vi "CSM - Synchronized Call.vi"   [LabVIEW 2017, in "CSM-QuickDrops.lvlib"]
doc: "Code snippet for calling a CSM module synchronously. This VI calls CSM module directly as a subVI.\n\n<b>Reference Example</b>: `[CSM-Example]\\2. Caller is CSM Scenario\\CSM Example - Caller is a CSM.vi`."
uses:
  CSM-QuickDrops.lvlib
  Communicable State Machine.lvlib
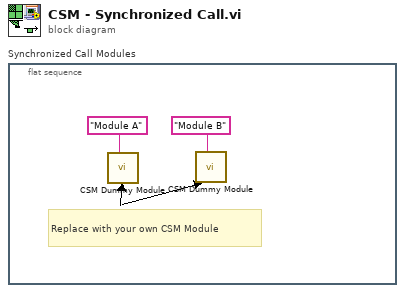
[diagram p0: block diagram]
diagram:
  n1 = flat-sequence "Synchronized Call Modules" {
    frame #0 {
      # "Replace with your own CSM Module"
      n2 = call "CSM Dummy Module.vi"("Name (\"\" to Use UUID)"="Module A" ("Name (\"\" to Use UUID)")) -> ()  [unwired: 11 in]
      n3 = call "CSM Dummy Module.vi"("Name (\"\" to Use UUID)"="Module B" ("Name (\"\" to Use UUID)")) -> ()  [unwired: 11 in]
    }
  }
